vi "diode.vi"() -> ()   [LabVIEW 2025]
uses:
  <vilib>/Utility/file.llb/Write Delimited Spreadsheet (DBL).vi
panel:
  out "XY Graph":cluster{dbl[], dbl[]}(graph)
  out "I":dbl(graph)
  out "AI":dbl(graph)
  out "AO":dbl(graph)
  in  "V_Stop":dbl
  in  "V_Start":dbl
  out "task out":refnum<k21>
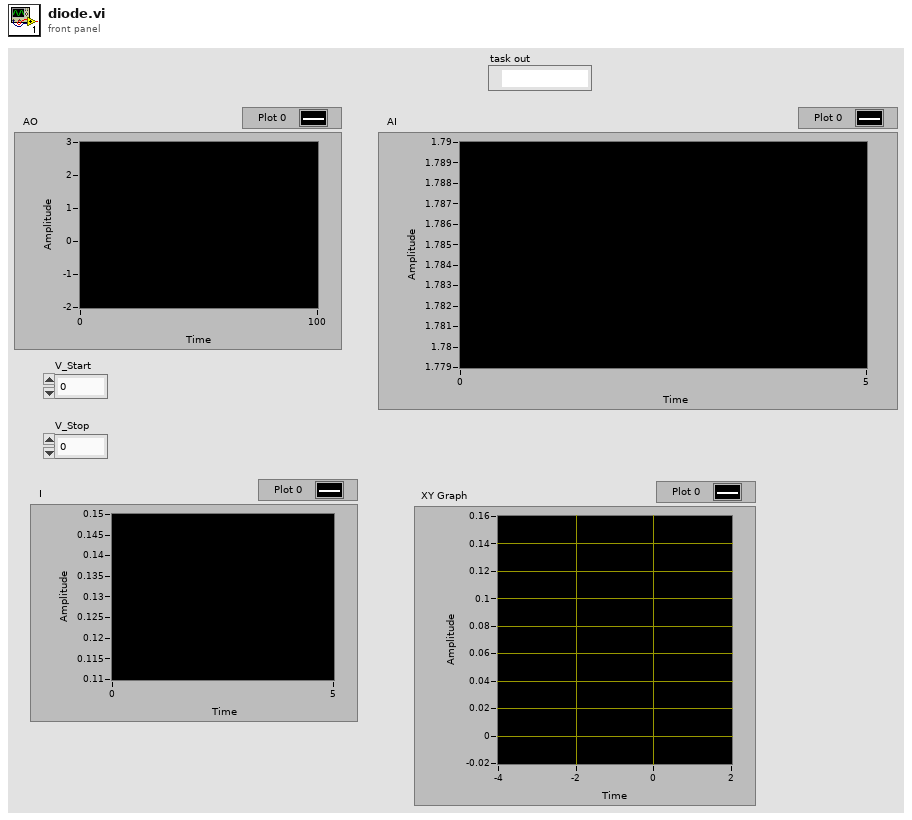
[diagram p1: front panel]
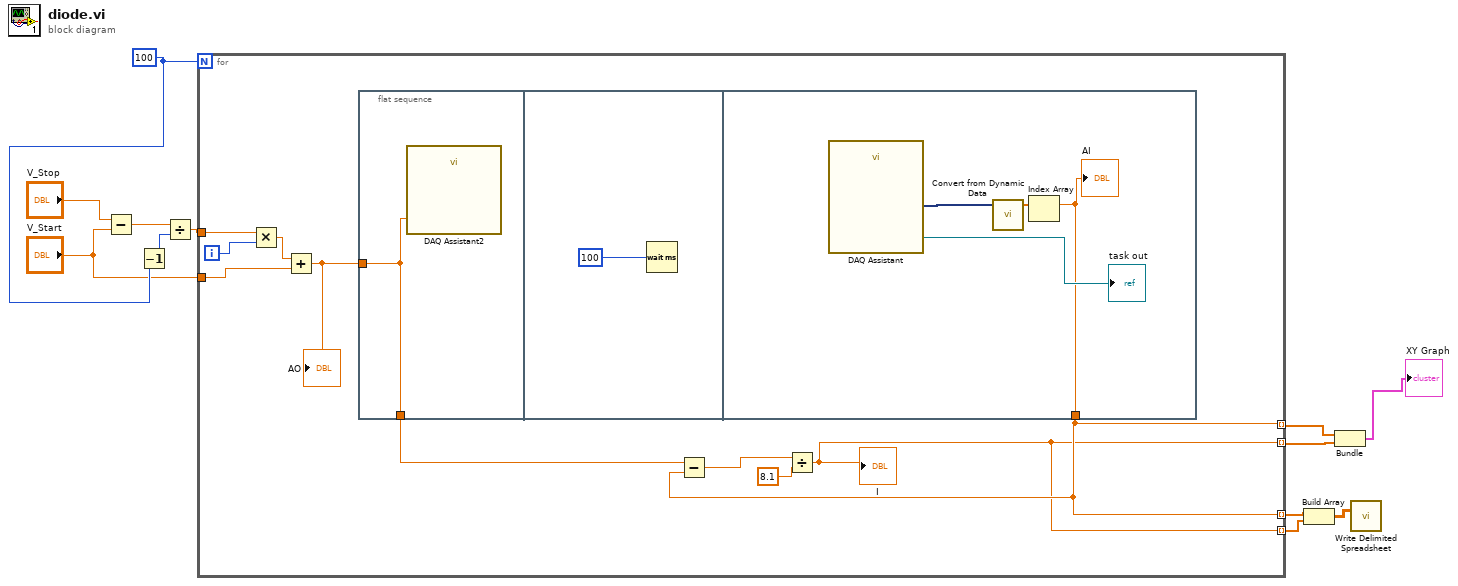
[diagram p0: block diagram]
diagram:
  w10 = 100
  n1 = Subtract(x="V_Stop", y="V_Start") -> (x-y=w11:dbl)
  n2 = Decrement(x=w10) -> (x-1=w9:i32)
  n3 = Divide(x=w11, y=w9) -> (x/y=w8:dbl)
  n4 = for {
    N: w10 -> [_]
    tunnel: w8 -> [w22]
    tunnel: "V_Start" -> [w19]
    tunnel: [w13] -> w5 mode=indexing
    tunnel: [w14] -> w6 mode=indexing
    tunnel: [w14] -> w3 mode=indexing
    tunnel: [w13] -> w2 mode=indexing
    i -> [w21]
    n5 = Multiply(x=w22, y=w21) -> (x*y=w20:dbl)
    n6 = Add(x=w20, y=w19) -> (x+y=w18:dbl)
    "AO" <- w18
    n7 = flat-sequence {
      tunnel: w18 -> [w23]
      tunnel: [w23] -> w17
      tunnel: [w26] -> w14
      frame #0 {
        n8 = call "DAQ Assistant2"("data"=w23) -> ()  [unwired: 17 in, 2 out]
      }
      frame #1 {
        n9 = Wait (ms)(milliseconds to wait=100) -> ()  [unwired: 1 out]
      }
      frame #2 {
        n10 = call "DAQ Assistant"() -> ("task out"=→"task out":refnum<k21>, "data"=w27:dynamicdata)  [unwired: 17 in, 1 out]
        n11 = call "Convert from Dynamic Data"("Dynamic Data Type"=w27) -> ("Array"=w25:dbl[])  [unwired: 3 in]
        n12 = Index Array(array=w25) -> (element=w26:dbl)  [unwired: 1 in]
        "AI" <- w26
      }
    }
    n13 = Subtract(x=w17, y=w14) -> (x-y=w16:dbl)
    n14 = Divide(x=w16, y=8.1) -> (x/y=w13:dbl)
    "I" <- w13
  }
  n15 = Build Array(w3, w2) -> (w1:dbl[][])
  n16 = Bundle(w6, w5) -> (→"XY Graph":cluster{dbl[], dbl[]})  [unwired: 1 in]
  n17 = call-poly <vilib>:"Write Delimited Spreadsheet.vi"("2D data"=w1) -> ()  [unwired: 13 in, 2 out]
